vi "Ortalama.vi"(3 "Array":sgl[](array[numeric])) -> (1 "Numeric":sgl)   [LabVIEW 2014]
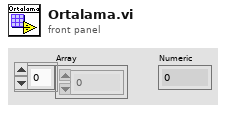
[diagram p1: front panel]
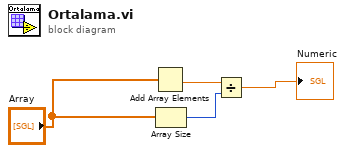
[diagram p0: block diagram]
diagram:
  n1 = Add Array Elements(numeric array="Array") -> (sum=w1:sgl)
  n2 = Array Size(array="Array") -> (size(s)=w3:i32)
  n3 = Divide(x=w1, y=w3) -> (x/y=→"Numeric":sgl)
